vi "orbit and angle panel.vi"() -> ()   [LabVIEW 2017]
uses:
  control panel globals.vi
panel:
  in  "clear slope and mag data":bool
  out "error out":errorcluster
  in  "time axis in hrs":bool=TRUE
  in  "hours of data to fit/display":dbl=5.0
  out "minor axis vs angle":cluster{dbl[], dbl[]}[](graph)
  out "minor axis vs time":cluster{dbl[], sgl[]}(graph)
  out "ellipse fit":T1
  out "orbit is":enum16{"clockwise", "counterclockwise"}(ring)
  out "deg/hr":dbl format="%0.2f"
  out "angle":dbl
  out "angle vs time":cluster{dbl[], dbl[]}[](graph)
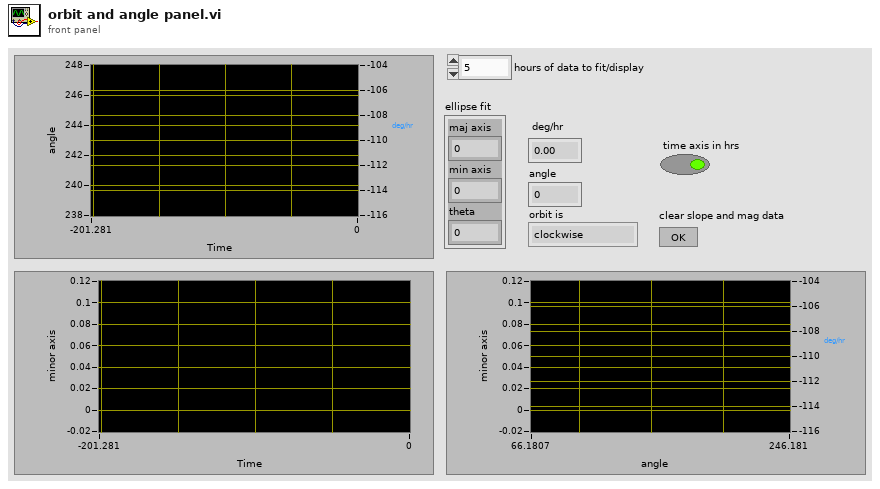
[diagram p1: front panel]
types:
  T1 = cluster{"maj axis":dbl, "min axis":dbl, "theta":dbl}
  T2 = typedef "queue cluster.ctl" = cluster{"voltage":T3, "coil":T3, "mag":T3, "accel":T3, "slope":T4, "angle":T3}
  T3 = typedef "reading queue.ctl" = refnum<queue>
  T4 = typedef "reading 1 queue.ctl" = refnum<queue>
  T5 = typedef "reading.ctl" = cluster{"reading type":T6, "time":fxp<+,48,48>, "x":sgl, "y":sgl, "z":sgl, "XSUM":u8}
  T6 = typedef "readingType.ctl" = enum8{"SYNC", "DETVAL", "COILI", "MAGVEC", "ACCVEC"}
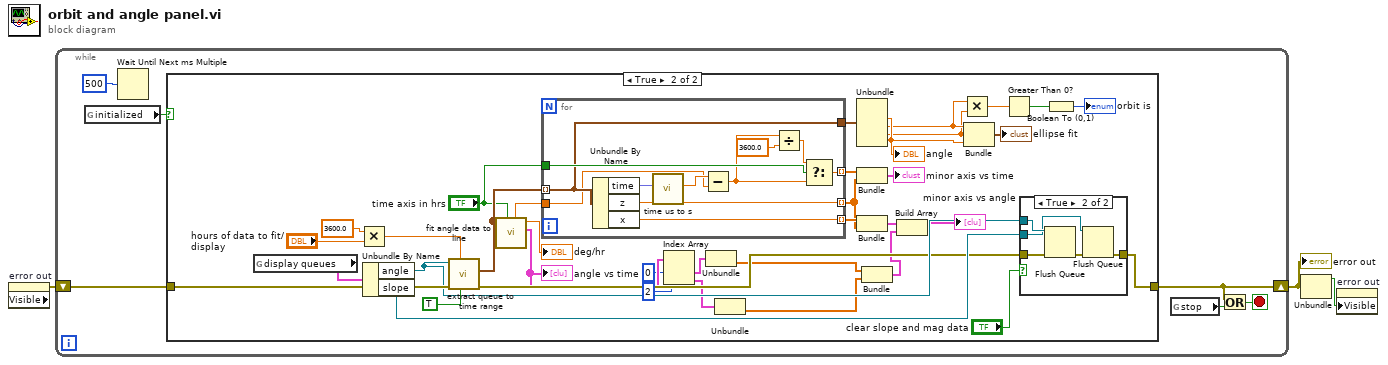
[diagram p0: block diagram]
diagram:
  n1 = property on="error out" class="Clust (strict)" props=["Visible"]() -> (error out=w1:errorcluster)  [unwired: 2 in, 2 out]
  n2 = while {
    shift-right: [w6] -> w3
    shift-left: w1 -> [w7]
    stop <- w4 stop-if-true
    n3 = global read "control panel globals.vi" "initialized"() -> (w9:bool)
    n4 = Wait Until Next ms Multiple(millisecond multiple=u32 500) -> ()  [unwired: 1 out]
    n5 = case shown="True" w9 {
      tunnel: [w10 w20] -> w6
      tunnel: w7 -> [w10 w26]
      frame False {
      }
      frame True {
        n6 = global read "control panel globals.vi" "display queues"() -> (w47:T2)
        n7 = Multiply(x=3600.0, y="hours of data to fit/display") -> (x*y=w45:dbl)
        n8 = Unbundle By Name(w47) -> ("angle"=w24:T3, "slope"=w23:T4)
        n9 = call "extract queue to time range.vi"("most recent?"=TRUE, "recent interval"=w45, "error in (no error)"=w26, "queue"=w24) -> ("error out"=w21:errorcluster, "extracted data"=w41:T5[])  [unwired: 6 in]
        n10 = call "fit angle data to line.vi"("hrs"="time axis in hrs", "remaining elements"=w41) -> ("graphs"=w19:cluster{dbl[], dbl[]}[], "deg/hr"=→"deg/hr":dbl, "tmax"=w25:dbl)  [unwired: 7 in]
        "angle vs time" <- w19
        n11 = for {
          tunnel: w41 -> [w56] mode=indexing
          tunnel: "time axis in hrs" -> [w61]
          tunnel: [w59] -> w39 mode=indexing
          tunnel: [w58] -> w36 mode=indexing
          tunnel: [w57] -> w37 mode=indexing
          tunnel: [w56] -> w34
          tunnel: w25 -> [w54]
          n12 = Unbundle By Name(w56) -> ("time"=w64:fxp<+,48,48>, "z"=w58:sgl, "x"=w57:sgl)
          n13 = call "time us to s.vi"("time (us)"=w64) -> ("time (s)"=w60:dbl)  [unwired: 10 in]
          n14 = Subtract(x=w60, y=w54) -> (x-y=w55:dbl)
          n15 = Divide(x=w55, y=3600.0) -> (x/y=w62:dbl)
          n16 = Select(t=w62, s=w61, f=w55) -> (s? t:f=w59:dbl)
        }
        n17 = Index Array(array=w19, index #1=0 ("index"), index #2=2 ("index")) -> (element #1=w16:cluster{dbl[], dbl[]}, element #2=w15:cluster{dbl[], dbl[]})
        n18 = Unbundle(w16) -> (w13:dbl[])  [unwired: 1 out]
        n19 = Unbundle(w15) -> (w14:dbl[])  [unwired: 1 out]
        n20 = Unbundle(w34) -> ("x"=w32:sgl, "y"=w31:sgl, "z"=w30:sgl)  [unwired: 3 out]
        "angle" <- w32
        n21 = Bundle(w39, w36) -> (→"minor axis vs time":cluster{dbl[], sgl[]})  [unwired: 1 in]
        n22 = Bundle(w37, w36) -> (w35:cluster{sgl[], sgl[]})  [unwired: 1 in]
        n23 = Bundle(w13, w14) -> (w11:cluster{dbl[], dbl[]})  [unwired: 1 in]
        n24 = Build Array(w35, w11) -> (→"minor axis vs angle":cluster{dbl[], dbl[]}[])
        n25 = Multiply(x=w31, y=w30) -> (x*y=w29:sgl)
        n26 = Bundle("y"=w31, "z"=w30, "x"=w32) -> (→"ellipse fit":cluster{"y":sgl, "z":sgl, "x":sgl})  [unwired: 1 in]
        n27 = Greater Than 0?(x=w29) -> (x > 0?=w28:bool)
        n28 = case shown="True" "clear slope and mag data" {
          tunnel: w21 -> [w48 w53]
          tunnel: [w48 w51] -> w20
          tunnel: w24 -> [_ w50]
          tunnel: w23 -> [_ w49]
          frame False {
          }
          frame True {
            n29 = Flush Queue(queue=w50, error in (no error)=w53) -> (error out=w52:errorcluster)  [unwired: 2 out]
            n30 = Flush Queue(queue=w49, error in (no error)=w52) -> (error out=w51:errorcluster)  [unwired: 2 out]
          }
        }
        n31 = Boolean To (0,1)(Boolean=w28) -> (0, 1=→"orbit is":i16)
      }
    }
    n32 = global read "control panel globals.vi" "stop"() -> (w5:bool)
    n33 = Or(x=w6, y=w5) -> (x .or. y?=w4:bool)
  }
  "error out" <- w3
  n34 = Unbundle(w3) -> ("status"=w2:bool)  [unwired: 2 out]
  n35 = property on="error out" class="Clust (strict)"("Visible"=w2) -> ()  [unwired: 2 in, 2 out]
